vi "Set RFPM Settings.vi"(0 "RFPM Handle In":refnum<k15>, 5 "RFPM Settings":T1 {"User-Defined Calibration"."Calibration Interval Check"."Calibration Interval (days)" format="%#_13g"; "User-Defined Calibration"."Calibration Interval Check"."Temperature Interval (deg C)" format="%#_13g"; "User-Defined Calibration"."Source Power Level Coercion Method" items=["Disabled"=1, "Nearest Power"=2, "Lower Power"=3]}, 11 "error in":errorcluster) -> (4 "RFPM Handle Out":refnum<k15>, 15 "error out":errorcluster)   [LabVIEW 2023, in "RFFixtureCharact.RFPM.lvlib" / "RF Subsystem Session Provider.lvclass"]
uses:
  RF Subsystem Session Provider.lvclass
  Controls/RFPM Settings.ctl
  Controls/Calibration Check.ctl
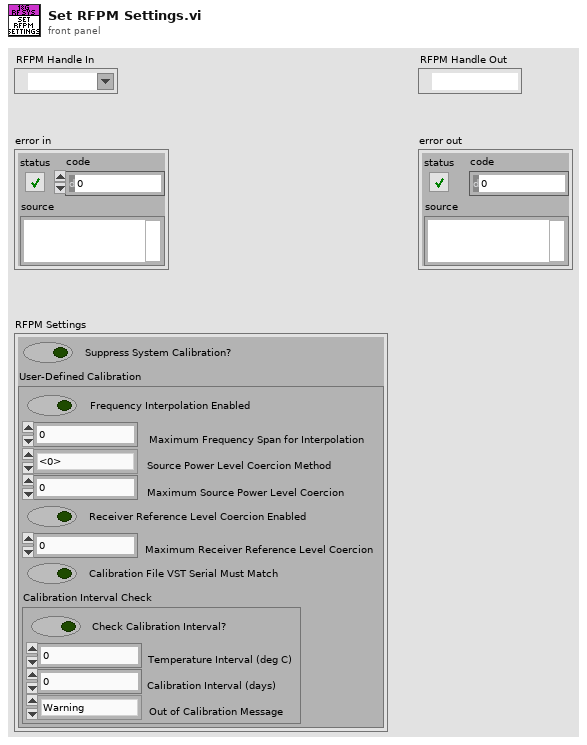
[diagram p1: front panel]
types:
  T1 = typedef "RFFixtureCharact.RFPM.lvlib/RF Subsystem Session Provider.lvclass/RFPM Settings.ctl" = cluster{"Suppress System Calibration?":bool, "User-Defined Calibration":cluster{"Frequency Interpolation Enabled":bool, "Maximum Frequency Span for Interpolation":dbl, "Source Power Level Coercion Method":i32, "Maximum Source Power Level Coercion":dbl, "Receiver Reference Level Coercion Enabled":bool, "Maximum Receiver Reference Level Coercion":dbl, "Calibration File VST Serial Must Match":bool, "Calibration Interval Check":T2}}
  T2 = typedef "RFFixtureCharact.RFPM.lvlib/RF Subsystem Session Provider.lvclass/Calibration Check.ctl" = cluster{"Check Calibration Interval?":bool, "Temperature Interval (deg C)":dbl, "Calibration Interval (days)":dbl, "Out of Calibration Message":enum16{"Warning", "Error"}}
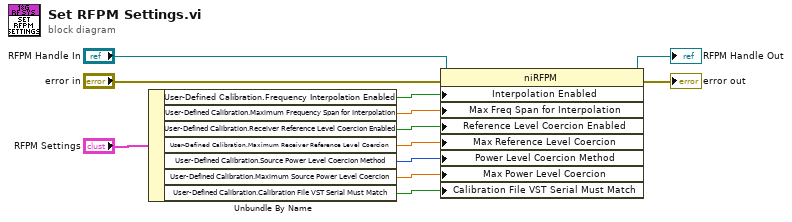
[diagram p0: block diagram]
diagram:
  n1 = Unbundle By Name("RFPM Settings") -> ("User-Defined Calibration.Frequency Interpolation Enabled"=w7:bool, "User-Defined Calibration.Maximum Frequency Span for Interpolation"=w6:dbl, "User-Defined Calibration.Receiver Reference Level Coercion Enabled"=w5:bool, "User-Defined Calibration.Maximum Receiver Reference Level Coercion"=w4:dbl, "User-Defined Calibration.Source Power Level Coercion Method"=w3:i32, "User-Defined Calibration.Maximum Source Power Level Coercion"=w2:dbl, "User-Defined Calibration.Calibration File VST Serial Must Match"=w1:bool)
  n2 = property class="niRFPM"(reference="RFPM Handle In", error in="error in", "Interpolation Enabled"=w7, "Max Freq Span for Interpolation"=w6, "Reference Level Coercion Enabled"=w5, "Max Reference Level Coercion"=w4, "Power Level Coercion Method"=w3, "Max Power Level Coercion"=w2, "Calibration File VST Serial Must Match"=w1) -> (reference out=→"RFPM Handle Out":refnum<k15>, error out=→"error out":errorcluster)
